vi "Collect.vi"(8 "error in (no error)":errorcluster, 11 "Default Collector in":refnum<class "Default Collector.lvclass">) -> (0 "error out":errorcluster, 2 "Metrics":refnum<data-value>[](array[refnum]), 3 "Default Collector out":refnum<class "Default Collector.lvclass">)   [LabVIEW 2020, in "Collector.lvlib" / "Default Collector.lvclass"]
uses:
  Default Collector.lvclass
  metrics/metric/Metric.lvclass
  Default Collector.lvclass/Default Collector.ctl
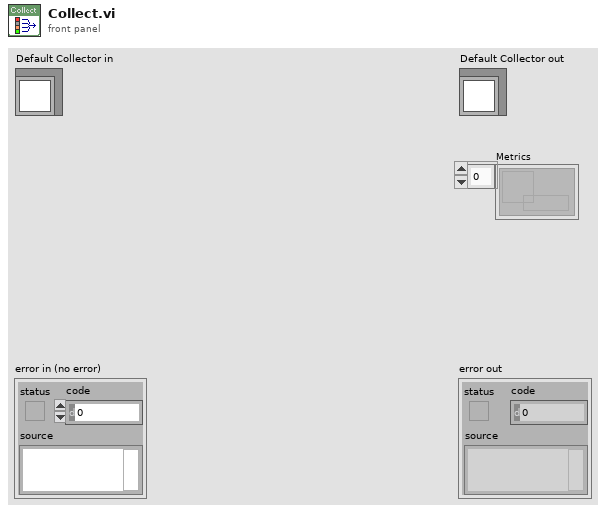
[diagram p1: front panel]
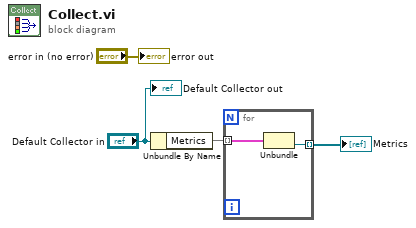
[diagram p0: block diagram]
diagram:
  n1 = Unbundle By Name("Default Collector in") -> ("Metrics"=w3:map{string, refnum<data-value>})
  n2 = for {
    tunnel: w3 -> [w6] mode=indexing
    tunnel: [w5] -> w2 mode=indexing
    n3 = Unbundle(w6) -> ("Metric"=w5:refnum<data-value>)  [unwired: 1 out]
  }
  "Metrics" <- w2
  "error out" <- "error in (no error)"
  "Default Collector out" <- "Default Collector in"
